vi "operate.vi"(9 "a to b":string, 10 "b":string, 11 "a":string) -> (3 "Result":string)   [LabVIEW 2020]
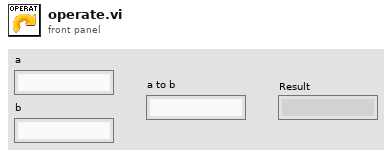
[diagram p1: front panel]
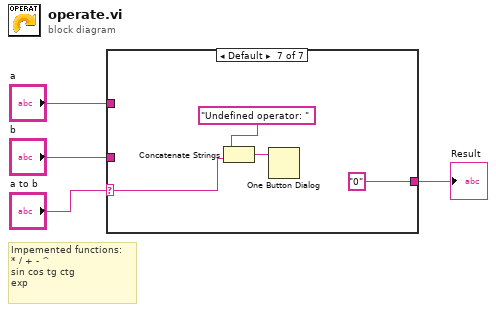
[diagram p0: block diagram]
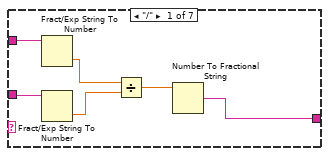
[diagram p2: hidden frame]
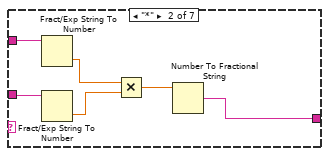
[diagram p3: hidden frame]
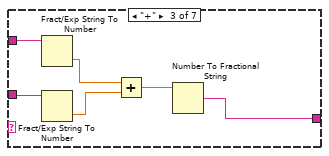
[diagram p4: hidden frame]
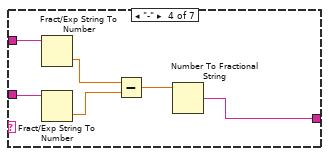
[diagram p5: hidden frame]
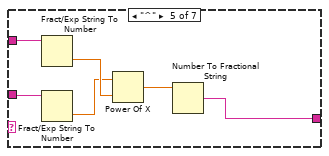
[diagram p6: hidden frame]
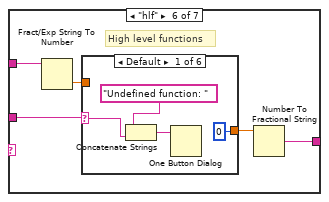
[diagram p7: hidden frame]
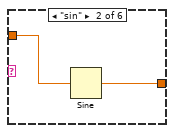
[diagram p8: hidden frame]
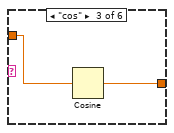
[diagram p9: hidden frame]
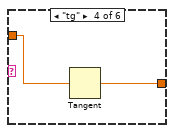
[diagram p10: hidden frame]
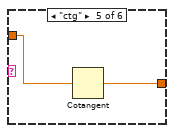
[diagram p11: hidden frame]
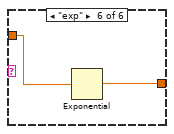
[diagram p12: hidden frame]
diagram:
  # "Impemented functions:\n* / + - ^\nsin cos tg ctg\nexp"
  n1 = case shown="Default" "a to b" {
    selector: "a to b" -> [_ _ _ _ _ _ w54]
    tunnel: "b" -> [w9 w15 w21 w27 w33 w37 _]
    tunnel: "a" -> [w10 w16 w22 w28 w34 w39 _]
    tunnel: [w5 w11 w17 w23 w32 w38 "0"] -> w1
    frame "/" {
      n2 = Fract/Exp String To Number(string=w10) -> (number=w8:dbl)  [unwired: 3 in, 1 out]
      n3 = Fract/Exp String To Number(string=w9) -> (number=w7:dbl)  [unwired: 3 in, 1 out]
      n4 = Divide(x=w8, y=w7) -> (x/y=w6:dbl)
      n5 = Number To Fractional String(number=w6) -> (F-format string=w5:string)  [unwired: 3 in]
    }
    frame "*" {
      n6 = Fract/Exp String To Number(string=w16) -> (number=w14:dbl)  [unwired: 3 in, 1 out]
      n7 = Fract/Exp String To Number(string=w15) -> (number=w13:dbl)  [unwired: 3 in, 1 out]
      n8 = Multiply(x=w14, y=w13) -> (x*y=w12:dbl)
      n9 = Number To Fractional String(number=w12) -> (F-format string=w11:string)  [unwired: 3 in]
    }
    frame "+" {
      n10 = Fract/Exp String To Number(string=w22) -> (number=w20:dbl)  [unwired: 3 in, 1 out]
      n11 = Fract/Exp String To Number(string=w21) -> (number=w19:dbl)  [unwired: 3 in, 1 out]
      n12 = Add(x=w20, y=w19) -> (x+y=w18:dbl)
      n13 = Number To Fractional String(number=w18) -> (F-format string=w17:string)  [unwired: 3 in]
    }
    frame "-" {
      n14 = Fract/Exp String To Number(string=w28) -> (number=w26:dbl)  [unwired: 3 in, 1 out]
      n15 = Fract/Exp String To Number(string=w27) -> (number=w25:dbl)  [unwired: 3 in, 1 out]
      n16 = Subtract(x=w26, y=w25) -> (x-y=w24:dbl)
      n17 = Number To Fractional String(number=w24) -> (F-format string=w23:string)  [unwired: 3 in]
    }
    frame "^" {
      n18 = Fract/Exp String To Number(string=w34) -> (number=w30:dbl)  [unwired: 3 in, 1 out]
      n19 = Fract/Exp String To Number(string=w33) -> (number=w29:dbl)  [unwired: 3 in, 1 out]
      n20 = Power Of X(1:w30, 2:w29) -> (0:w31:dbl)
      n21 = Number To Fractional String(number=w31) -> (F-format string=w32:string)  [unwired: 3 in]
    }
    frame "hlf" {
      # "High level functions"
      n22 = Fract/Exp String To Number(string=w39) -> (number=w35:dbl)  [unwired: 3 in, 1 out]
      n23 = case shown="Default" w37 {
        selector: w37 -> [w42 _ _ _ _ _]
        tunnel: [0 w44 w47 w49 w51 w53] -> w36
        tunnel: w35 -> [_ w45 w46 w48 w50 w52]
        frame Default {
          n24 = Concatenate Strings("Undefined function: ", w42) -> (w41:string)
          n25 = One Button Dialog(message=w41) -> ()  [unwired: 1 in, 1 out]
        }
        frame "sin" {
          n26 = Sine(x=w45) -> (sin(x)=w44:dbl)
        }
        frame "cos" {
          n27 = Cosine(x=w46) -> (cos(x)=w47:dbl)
        }
        frame "tg" {
          n28 = Tangent(1:w48) -> (0:w49:dbl)
        }
        frame "ctg" {
          n29 = Cotangent(1:w50) -> (0:w51:dbl)
        }
        frame "exp" {
          n30 = Exponential(1:w52) -> (0:w53:dbl)
        }
      }
      n31 = Number To Fractional String(number=w36) -> (F-format string=w38:string)  [unwired: 3 in]
    }
    frame Default {
      n32 = Concatenate Strings("Undefined operator: ", w54) -> (w55:string)
      n33 = One Button Dialog(message=w55) -> ()  [unwired: 1 in, 1 out]
    }
  }
  "Result" <- w1
